vi "Read Target.vi"(8 "error in (no error)":errorcluster, 11 "VeriStandScriptingTestCase in":refnum<class "VeriStandScriptingTestCase.lvclass">) -> (0 "error out":errorcluster, 2 "Target":refnum<k24>, 3 "VeriStandScriptingTestCase out":refnum<class "VeriStandScriptingTestCase.lvclass">)   [LabVIEW 2017, in "VeriStandScriptingTestCase.lvclass"]
uses:
  VeriStandScriptingTestCase.lvclass
  NationalInstruments.VeriStand.SystemDefinitionAPI
  VeriStandScriptingTestCase.lvclass/VeriStandScriptingTestCase.ctl
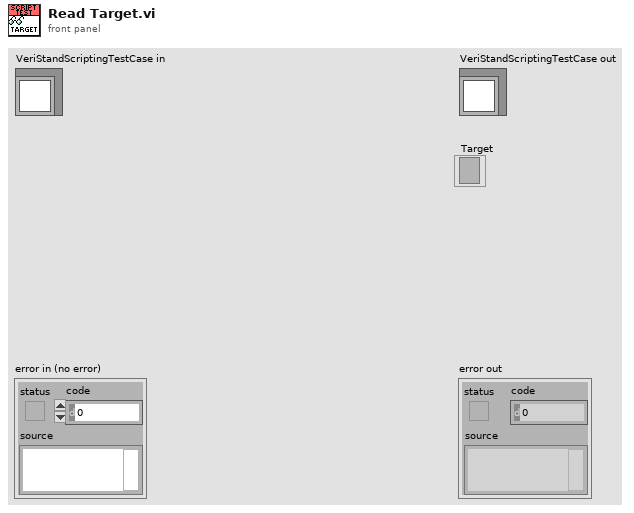
[diagram p1: front panel]
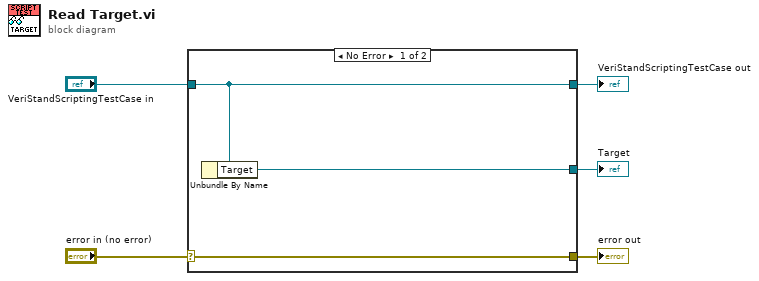
[diagram p0: block diagram]
diagram:
  n1 = case shown="No Error" "error in (no error)" {
    selector: "error in (no error)" -> [w8 w9]
    tunnel: [w8 w9] -> w4
    tunnel: [w7 w10] -> w2
    tunnel: "VeriStandScriptingTestCase in" -> [w7 w10]
    tunnel: [w6 _] -> w1
    frame No Error {
      n2 = Unbundle By Name(w7) -> ("Target"=w6:refnum<k24>)
    }
    frame Error {
    }
  }
  "error out" <- w4
  "VeriStandScriptingTestCase out" <- w2
  "Target" <- w1
